vi "double_temp.vi"(2 "V_2":fxp<+/-,24,5>, 3 "V_1":fxp<+/-,24,5>) -> (0 "T_2":i32, 1 "T_1":i32)   [LabVIEW 2018]
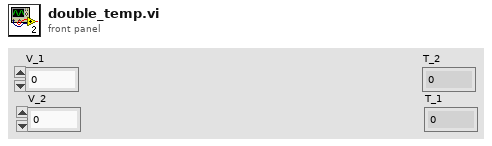
[diagram p1: front panel]
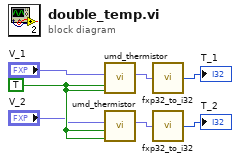
[diagram p0: block diagram]
diagram:
  w7 = TRUE
  n1 = call "umd_thermistor.vi"("ready for output (T)"=w7, "input valid"=w7, "V"="V_1") -> ("Temperature"=w4:fxp<+/-,32,16>)  [unwired: 7 in, 1 out]
  n2 = call "umd_thermistor.vi"("ready for output (T)"=w7, "input valid"=w7, "V"="V_2") -> ("Temperature"=w1:fxp<+/-,32,16>)  [unwired: 7 in, 1 out]
  n3 = call "fxp32_to_i32.vi"("fxp32_16"=w4) -> ("32bit integer"=→"T_1":i32)
  n4 = call "fxp32_to_i32.vi"("fxp32_16"=w1) -> ("32bit integer"=→"T_2":i32)
